vi "Read Channels.vi"(8 "error in (no error)":errorcluster, 11 "CryoCoolerAVC in":refnum<class "CryoCoolerAVC.lvclass">) -> (0 "error out":errorcluster, 2 "Channels":string[](array[string]), 3 "CryoCoolerAVC out":refnum<class "CryoCoolerAVC.lvclass">)   [LabVIEW 2022 SP3, in "CryoCoolerAVC.lvclass"]
uses:
  CryoCoolerAVC.lvclass
  CryoCoolerAVC.lvclass/CryoCoolerAVC.ctl
  Cryo Cooler.lvclass
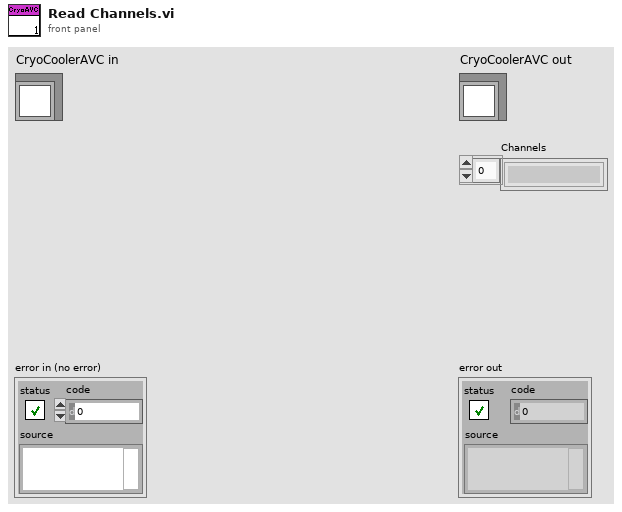
[diagram p1: front panel]
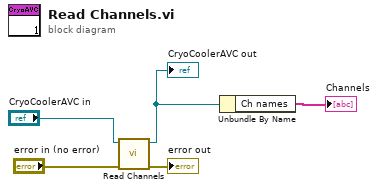
[diagram p0: block diagram]
diagram:
  n1 = call-parent "Read Channels.vi"("error in (no error)"="error in (no error)", "Cryo Cooler in"="CryoCoolerAVC in") -> ("error out"=→"error out":errorcluster, "Cryo Cooler out"=w2:refnum<class "CryoCoolerAVC.lvclass">)  [unwired: 7 in, 1 out]
  "CryoCoolerAVC out" <- w2
  n2 = Unbundle By Name(w2) -> ("Ch names"=→"Channels":string[])
